vi "Get Default Plugin Directories.vi"() -> (3 "Default Plugin Directories":path[](array[path]))   [LabVIEW 2020, in "RxnRover.lvlib" / "Plugin Manager.lvlib"]
uses:
  Plugin Manager.lvlib
  <vilib>/Utility/sysdir.llb/System Directory Type.ctl
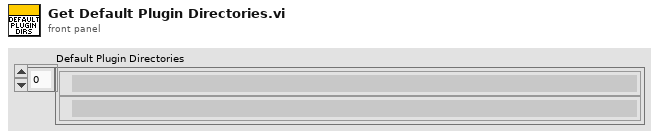
[diagram p1: front panel]
types:
  T1 = enum32{"invalid app kind", "Development System", "Run Time System", "Student Edition", "Embedded LabVIEW", "Evaluation", "Custom"}
  T2 = typedef "System Directory Type.ctl" = i32
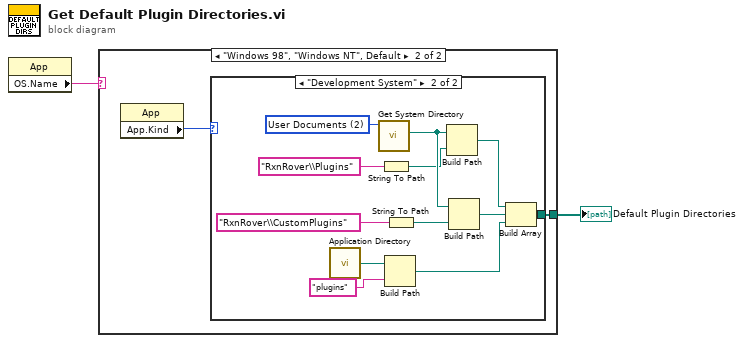
[diagram p0: block diagram]
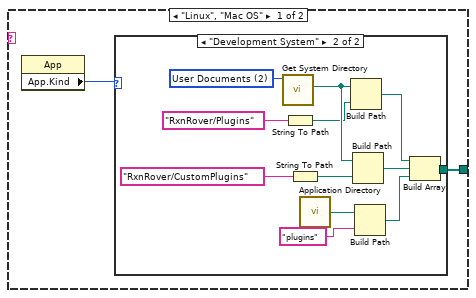
[diagram p2: hidden frame]
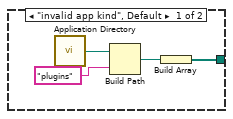
[diagram p3: hidden frame]
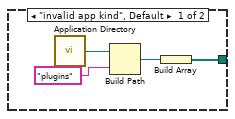
[diagram p4: hidden frame]
diagram:
  n1 = property class="App"() -> ("OS.Name"=w1:string)  [unwired: 2 in, 2 out]
  n2 = case shown="\"Windows 98\", \"Windows NT\", Default" w1 {
    tunnel: [w4 w22] -> w2
    frame "Linux", "Mac OS" {
      n3 = property class="App"() -> ("App.Kind"=w3:T1)  [unwired: 2 in, 2 out]
      n4 = case shown="\"Development System\"" w3 {
        tunnel: [w6 w12] -> w4
        frame "invalid app kind", Default {
          n5 = call <vilib>:"Application Directory.vi"() -> ("Application Directory"=w8:path)
          n6 = Build Path(base path=w8, name or relative path="plugins") -> (appended path=w5:path)
          n7 = Build Array(w5) -> (w6:path[])
        }
        frame "Development System" {
          w20 = T2 2 items=["User Home"=0, "User Desktop"=1, "User Documents"=2, "User Application Data"=3, "User Preferences"=4, "User Temporary"=5, "Public Documents"=6, "Public Application Data"=7, "Public Preferences"=8, "Public Cache"=13, "System Core Libraries"=9, "System Installed Libraries"=10, "Application Files"=11, "Boot Volume Root"=12] ("system directory type")
          n8 = call <vilib>:"Get System Directory.vi"("system directory type"=w20) -> ("system directory"=w18:path)  [unwired: 10 in]
          n9 = String To Path(string="RxnRover/Plugins" ("name or relative path")) -> (path=w14:path)
          n10 = String To Path(string="RxnRover/CustomPlugins" ("name or relative path")) -> (path=w13:path)
          n11 = call <vilib>:"Application Directory.vi"() -> ("Application Directory"=w11:path)
          n12 = Build Path(base path=w18, name or relative path=w14) -> (appended path=w17:path)
          n13 = Build Path(base path=w18, name or relative path=w13) -> (appended path=w16:path)
          n14 = Build Path(base path=w11, name or relative path="plugins") -> (appended path=w9:path)
          n15 = Build Array(w17, w16, w9) -> (w12:path[])
        }
      }
    }
    frame "Windows 98", "Windows NT", Default {
      n16 = property class="App"() -> ("App.Kind"=w21:T1)  [unwired: 2 in, 2 out]
      n17 = case shown="\"Development System\"" w21 {
        tunnel: [w23 w32] -> w22
        frame "invalid app kind", Default {
          n18 = call <vilib>:"Application Directory.vi"() -> ("Application Directory"=w26:path)
          n19 = Build Path(base path=w26, name or relative path="plugins") -> (appended path=w24:path)
          n20 = Build Array(w24) -> (w23:path[])
        }
        frame "Development System" {
          w38 = T2 2 items=["User Home"=0, "User Desktop"=1, "User Documents"=2, "User Application Data"=3, "User Preferences"=4, "User Temporary"=5, "Public Documents"=6, "Public Application Data"=7, "Public Preferences"=8, "Public Cache"=13, "System Core Libraries"=9, "System Installed Libraries"=10, "Application Files"=11, "Boot Volume Root"=12] ("system directory type")
          n21 = call <vilib>:"Application Directory.vi"() -> ("Application Directory"=w29:path)
          n22 = call <vilib>:"Get System Directory.vi"("system directory type"=w38) -> ("system directory"=w36:path)  [unwired: 10 in]
          n23 = String To Path(string="RxnRover\\Plugins" ("name or relative path")) -> (path=w31:path)
          n24 = Build Path(base path=w29, name or relative path="plugins") -> (appended path=w27:path)
          n25 = String To Path(string="RxnRover\\CustomPlugins" ("name or relative path")) -> (path=w30:path)
          n26 = Build Path(base path=w36, name or relative path=w31) -> (appended path=w35:path)
          n27 = Build Path(base path=w36, name or relative path=w30) -> (appended path=w34:path)
          n28 = Build Array(w35, w34, w27) -> (w32:path[])
        }
      }
    }
  }
  "Default Plugin Directories" <- w2
